vi "fgv_Err-Device.vi"(7 "Err Sel":T2(ring), 9 "first?":bool, 10 "cmd":T1=enum."open", 11 "error in":errorcluster) -> ()   [LabVIEW 2019]
uses:
  cmd_err.ctl
  _ctrl/rw.ctl
  _ctrl/init-r-stop.ctl
  _ctrl/system-status.ctl
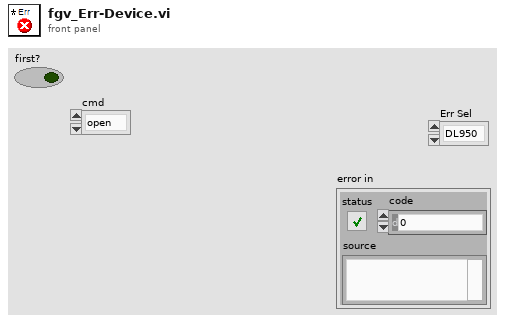
[diagram p1: front panel]
types:
  T1 = typedef "cmd_err.ctl" = enum16{"close", "open", "default"}
  T2 = enum16{"DL950", "BP4610", "DSP1500", "cDAQ-AI", "cDAQ-AO", "cDAQ-DO"}
  T3 = typedef "init-r-stop.ctl" = enum16{"ini", "read", "stop"}
  T4 = typedef "rw.ctl" = enum16{"read", "write"}
  T5 = typedef "Error list.ctl" = cluster{"DL950":bool, "BP4610":bool, "DSP":bool, "AI":bool, "AO":bool, "DO":bool}
  T6 = typedef "system-status.ctl" = enum16{"Initial", "Update", "Clear", "Read"}
  T7 = enum16{"clear", "Red", "Yellow", "Beep", "Beep onoff"}
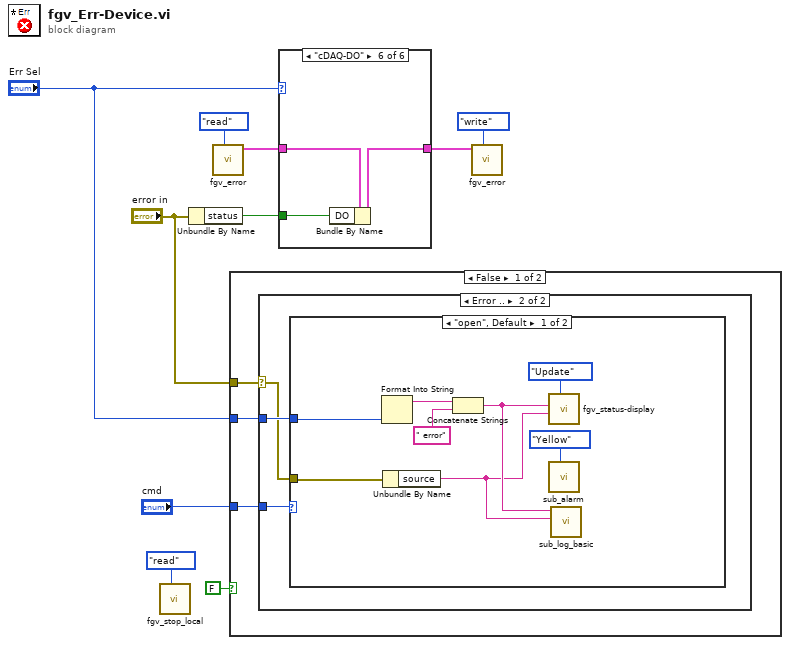
[diagram p0: block diagram]
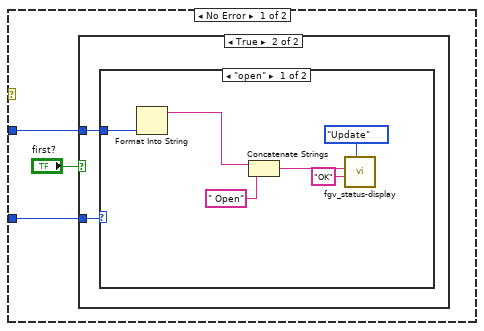
[diagram p2: hidden frame]
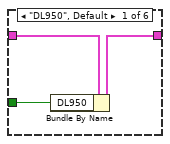
[diagram p7: hidden frame]
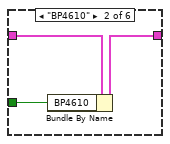
[diagram p8: hidden frame]
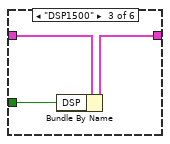
[diagram p9: hidden frame]
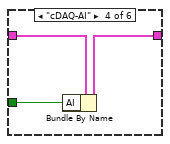
[diagram p10: hidden frame]
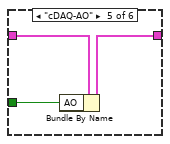
[diagram p11: hidden frame]
diagram:
  n1 = call "fgv_stop_local.vi"("cmd"=init-r-stop."read") -> ()  [unwired: 9 in, 2 out]
  n2 = Unbundle By Name("error in") -> ("status"=w6:bool)
  n3 = call "fgv_error.vi"("cmd"=rw."read") -> ("error cluster 2"=w8:T5)  [unwired: 9 in, 1 out]
  n4 = case shown="False" FALSE {
    tunnel: "Err Sel" -> [w13 _]
    tunnel: "error in" -> [w12 _]
    tunnel: "cmd" -> [w11 _]
    frame False {
      n5 = case shown="Error .." w12 {
        selector: w12 -> [_ w26]
        tunnel: w13 -> [w15 w27]
        tunnel: w11 -> [w16 w25]
        frame No Error {
          n6 = case shown="True" "first?" {
            tunnel: w16 -> [_ w18]
            tunnel: w15 -> [_ w17]
            frame False {
            }
            frame True {
              n7 = case shown="\"open\"" w18 {
                tunnel: w17 -> [w19 _]
                frame "open" {
                  n8 = Format Into String(w19) -> (resulting string=w23:string)  [unwired: 3 in, 1 out]
                  n9 = Concatenate Strings(w23, " Open" ("title")) -> (w24:string)
                  n10 = call "fgv_status-display.vi"("Mode"=system-status."Update", "detail"="OK", "title"=w24) -> ()  [unwired: 8 in, 1 out]
                }
                frame "close", Default {
                }
              }
            }
          }
        }
        frame Error {
          n11 = case shown="\"open\", Default" w25 {
            tunnel: w27 -> [w34 _]
            tunnel: w26 -> [w31 _]
            frame "open", Default {
              n12 = Format Into String(w34) -> (resulting string=w33:string)  [unwired: 3 in, 1 out]
              n13 = Unbundle By Name(w31) -> ("source"=w28:string)
              n14 = Concatenate Strings(w33, " error" ("title")) -> (w29:string)
              n15 = call "fgv_status-display.vi"("Mode"=system-status."Update", "detail"=w28, "title"=w29) -> ()  [unwired: 8 in, 1 out]
              n16 = call "sub_alarm.vi"("alarm"=T7."Yellow") -> ()  [unwired: 11 in]
              n17 = call "sub_log_basic.vi"("desc"=w28, "Title"=w29) -> ()  [unwired: 9 in, 1 out]
            }
            frame "close" {
            }
          }
        }
      }
    }
    frame True {
    }
  }
  n18 = case shown="\"cDAQ-DO\"" "Err Sel" {
    tunnel: w6 -> [w38 w41 w44 w47 w50 w53]
    tunnel: w8 -> [w37 w40 w43 w46 w49 w52]
    tunnel: [w36 w39 w42 w45 w48 w51] -> w7
    frame "DL950", Default {
      n19 = Bundle By Name(cluster=w37, "DL950"=w38) -> (w36:T5)
    }
    frame "BP4610" {
      n20 = Bundle By Name(cluster=w40, "BP4610"=w41) -> (w39:T5)
    }
    frame "DSP1500" {
      n21 = Bundle By Name(cluster=w43, "DSP"=w44) -> (w42:T5)
    }
    frame "cDAQ-AI" {
      n22 = Bundle By Name(cluster=w46, "AI"=w47) -> (w45:T5)
    }
    frame "cDAQ-AO" {
      n23 = Bundle By Name(cluster=w49, "AO"=w50) -> (w48:T5)
    }
    frame "cDAQ-DO" {
      n24 = Bundle By Name(cluster=w52, "DO"=w53) -> (w51:T5)
    }
  }
  n25 = call "fgv_error.vi"("cmd"=rw."write", "error cluster"=w7) -> ()  [unwired: 8 in, 2 out]
